vi "字符串数组除空白1.vi"(8 "error in (no error)":errorcluster caption="错误输入（无错误）", 11 "输入字符串数组":string[](array[string])) -> (0 "错误输出":errorcluster, 3 "输出字符串数组":string[](array[string]))   [LabVIEW 2018]
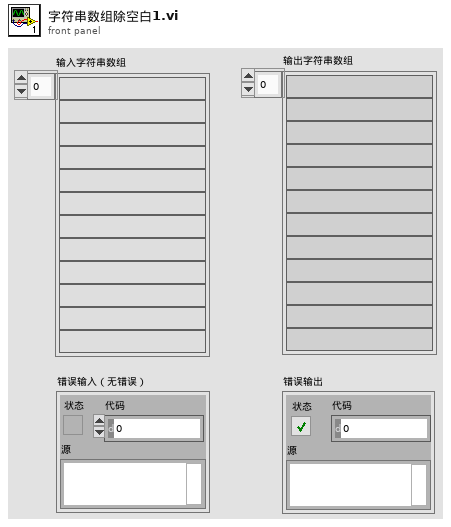
[diagram p1: front panel]
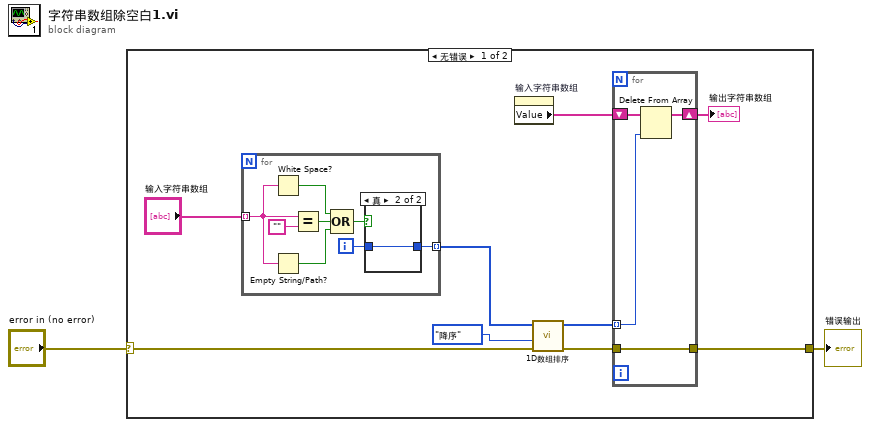
[diagram p0: block diagram]
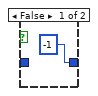
[diagram p2: hidden frame]
diagram:
  n1 = case shown="无错误" "error in (no error)" {
    selector: "error in (no error)" -> [w7 w26]
    tunnel: [w6 w26] -> w1
    frame No Error {
      n2 = for {
        tunnel: "输入字符串数组" -> [w20] mode=indexing
        tunnel: [w22] -> w11 mode=indexing
        i -> [w23]
        n3 = White Space?(1:w20) -> (0:w19:bool)
        n4 = Empty String/Path?(string/path=w20) -> (empty?=w17:bool)
        n5 = Equal?(x=w20, y="") -> (x = y?=w18:bool)
        n6 = Compound Arithmetic op=OR(w19, w18, w17) -> (w16:bool)
        n7 = case shown="真" w16 {
          tunnel: w23 -> [_ w25]
          tunnel: [-1 w25] -> w22
          frame False {
          }
          frame True {
          }
        }
      }
      n8 = property on="输入字符串数组" class="Arr (严格)"() -> ("Value"=w4:string[])  [unwired: 2 in, 2 out]
      n9 = call-poly "1D数组排序.vi"("error in (no error)"=w7, "升降序"=enum16{"升序", "降序"}."降序", "输入数组"=w11) -> ("error out"=w8:errorcluster, "排序后数组"=w9:i32[])  [unwired: 6 in, 1 out]
      n10 = for {
        tunnel: w9 -> [w15] mode=indexing
        tunnel: w8 -> [w14]
        tunnel: [w14] -> w6
        shift-right: [w12] -> w3
        shift-left: w4 -> [w13]
        n11 = Delete From Array(array=w13, index=w15) -> (array with subset deleted=w12:string[])  [unwired: 1 in, 1 out]
      }
      "输出字符串数组" <- w3
    }
    frame Error {
    }
  }
  "错误输出" <- w1
